vi "HTTP_REPL_Read.vi"(8 "error in (no error)":errorcluster, 11 "Clear":bool) -> (0 "error out":errorcluster, 2 "GET Code":T1, 3 "REPL":string)   [LabVIEW 2020]
uses:
  RestAPI.ctl
  JSON_Formats.vi
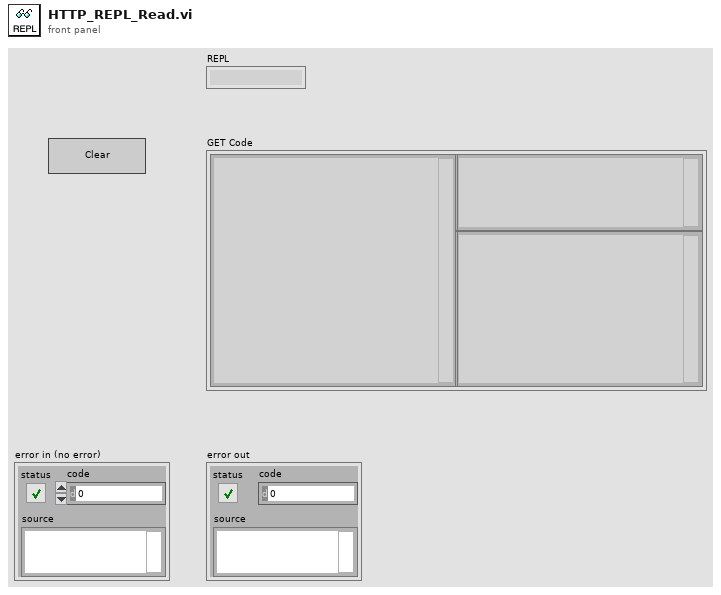
[diagram p1: front panel]
types:
  T1 = typedef "RestAPI.ctl" = cluster{"headers 2":string, "headers":string, "body":string}
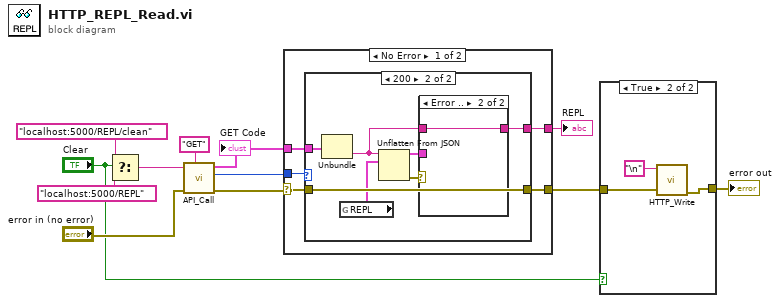
[diagram p0: block diagram]
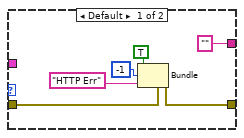
[diagram p3: hidden frame]
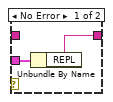
[diagram p4: hidden frame]
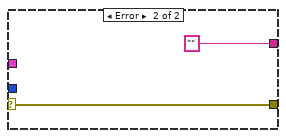
[diagram p5: hidden frame]
diagram:
  n1 = Select(t="localhost:5000/REPL/clean" ("url"), s="Clear", f="localhost:5000/REPL" ("url")) -> (s? t:f=w4:string)
  n2 = call "API_Call.vi"("Cmd"="GET" ("input 1"), "error in (no error)"="error in (no error)", "url"=w4) -> ("error out"=w10:errorcluster, "Err Code"=w9:i32, "Communication"=w11:T1)  [unwired: 6 in]
  "GET Code" <- w11
  n3 = case shown="No Error" w10 {
    selector: w10 -> [w16 w35]
    tunnel: w9 -> [w17 _]
    tunnel: [w15 w35] -> w2
    tunnel: w11 -> [w14 _]
    tunnel: [w13 "" ("REPL")] -> w12
    frame No Error {
      n4 = case shown="200" w17 {
        tunnel: w16 -> [w23 w30]
        tunnel: [w22 w30] -> w15
        tunnel: w14 -> [_ w29]
        tunnel: ["" ("REPL") w26] -> w13
        frame Default {
          n5 = Bundle(cluster=w23, "status"=TRUE, "code"=-1, "source"="HTTP Err") -> (w22:errorcluster)
        }
        frame 200 {
          n6 = Unbundle(w29) -> ("body"=w24:string)  [unwired: 2 out]
          n7 = global read "JSON_Formats.vi" "REPL"() -> (w28:cluster{"REPL":string})
          n8 = Unflatten From JSON(JSON string=w24, type and defaults=w28) -> (value=w27:cluster{"REPL":string}, error out=w25:errorcluster)  [unwired: 5 in]
          n9 = case shown="Error .." w25 {
            tunnel: w27 -> [w32 _]
            tunnel: [w31 w33] -> w26
            tunnel: w24 -> [_ w33]
            frame No Error {
              n10 = Unbundle By Name(w32) -> ("REPL"=w31:string)
            }
            frame Error {
            }
          }
        }
      }
    }
    frame Error {
    }
  }
  "REPL" <- w12
  n11 = case shown="True" "Clear" {
    tunnel: w2 -> [w36 w38]
    tunnel: [w36 w37] -> w1
    frame False {
    }
    frame True {
      n12 = call "HTTP_Write.vi"("error in (no error)"=w38, "Code"="\n") -> ("error out"=w37:errorcluster)  [unwired: 8 in, 1 out]
    }
  }
  "error out" <- w1
